vi "camera acquire test.vi"() -> ()   [LabVIEW 2014]
uses:
  SubVIs/ctt's/Image size and binning.ctl
  SubVIs/ctt's/Camera Setup Acquisition.ctl
panel:
  in  "EM CCD Gain":u16(slide)=300 scale=0.01..300.0
  in  "Acquisition Parameters":T1={"Set Acquisition Mode"=enum."Run till abort", "Trigger Mode"=enum."Internal", "Set VS Speed"=6.5, "Pixel Rate"=enum."EM CCD 5 Mhz 14 bits", "V Shift Amplitude"=enum."normal", "Readout Mode"=enum."Image", "Single Track \nSettings"={"centre"=0, "height"=1}, "Preamp Gain"=enum."2.4", "Number of\nAccumulations"=1, "Number of Kinetics"=1, "Accumulation\nCycle (s)"=1.0, "Kinetic Cycle Time (s)"=0.0, "High Capacity?"=FALSE} {"Single Track \nSettings"."centre" min=0 max=1024; "Single Track \nSettings"."height" min=1 max=1024; "Set VS Speed" min=0.0 format="%#_2f"}
  in  "Image Size":T2 {"V Bin" min=0.0; "H Bin" min=0.0 step=1.0}
  out "Error Out":errorcluster
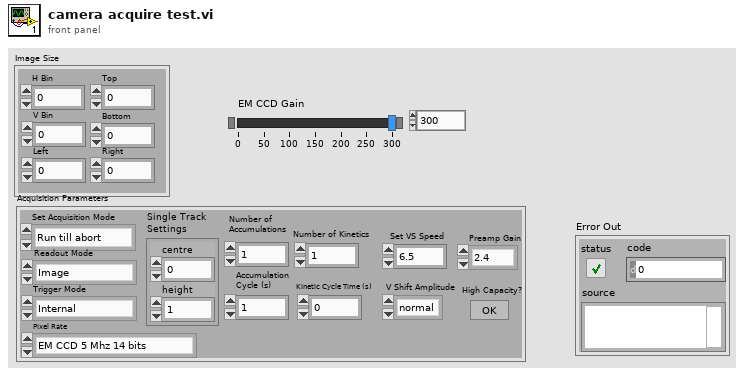
[diagram p1: front panel]
types:
  T1 = typedef "Camera Setup Acquisition.ctl" = cluster{"Set Acquisition Mode":enum16{"(do nothing)", "Single Scan", "Accumulate", "Kinetics", "Fast Kinetics", "Run till abort"}, "Trigger Mode":enum16{"Internal", "External"}, "Set VS Speed":dbl, "Pixel Rate":enum16{"EM CCD 10 Mhz 14 bits", "EM CCD 5 Mhz 14 bits", "EM CCD 3 Mhz 14 bits", "EM CCD 1 Mhz 16 bits", "Standard CCD 3 Mhz 14 bits", "Standard CCD 1 Mhz 16 bits"}, "V Shift Amplitude":enum16{"normal", "+1", "+2", "+3", "+4"}, "Readout Mode":enum16{"Full Vertical Binning", "Multi-Track", "Random-Track", "Single-Track", "Image"}, "Single Track \nSettings":cluster{"centre":i32, "height":i32}, "Preamp Gain":enum16{"1.0", "2.4", "5.0"}, "Number of\nAccumulations":i32, "Number of Kinetics":i32, "Accumulation\nCycle (s)":dbl, "Kinetic Cycle Time (s)":dbl, "High Capacity?":bool}
  T2 = typedef "Image size and binning.ctl" = cluster{"H Bin":dbl, "V Bin":dbl, "Left":dbl, "Right":dbl, "Top":dbl, "Bottom":dbl}
  T3 = typedef "Image Type" = u32
  T4 = typedef "IMAQ Image.ctl" = refnum<image>
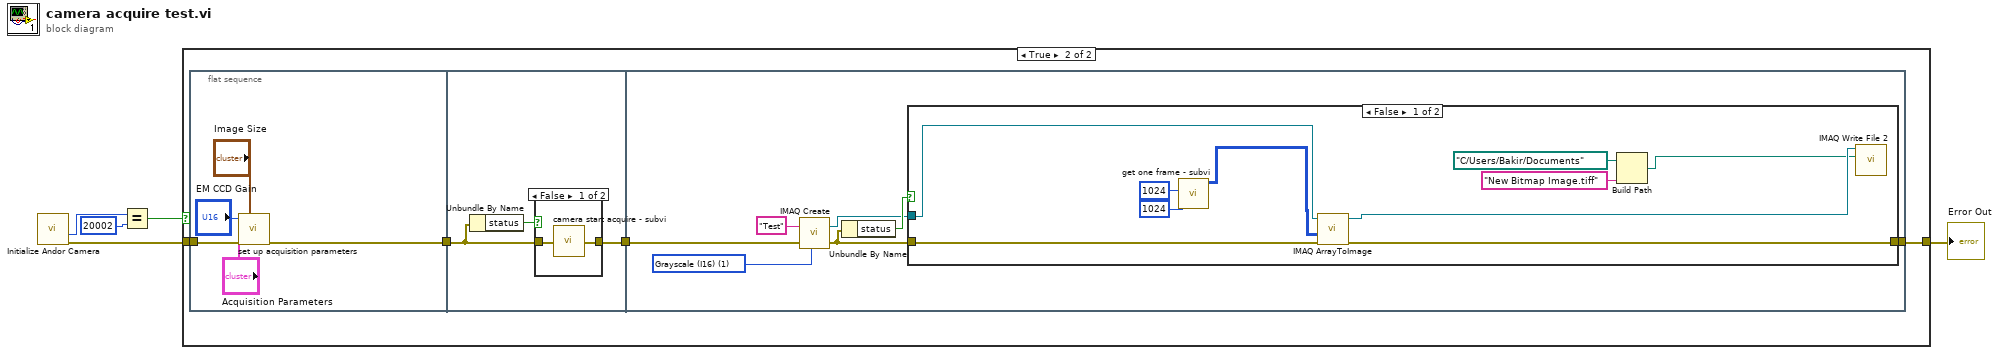
[diagram p0: block diagram]
diagram:
  n1 = call "Initialize Andor Camera.vi"() -> ("Error Out 2"=w4:errorcluster, "Drv Success?"=w1:i32)  [unwired: 10 in]
  n2 = Equal?(x=w1, y=20002) -> (x = y?=w3:bool)
  n3 = case shown="True" w3 {
    tunnel: [w6 w8] -> w5
    tunnel: w4 -> [w6 w7]
    frame False {
    }
    frame True {
      n4 = flat-sequence {
        tunnel: [w14] -> w10
        tunnel: w7 -> [w15]
        tunnel: w10 -> [w17]
        tunnel: [w16] -> w9
        tunnel: w9 -> [w25]
        tunnel: [w22] -> w8
        frame #0 {
          n5 = call "set up acquisition parameters.vi"("error in (no error)"=w15, "Acquisition Parameters"="Acquisition Parameters", "Image Size"="Image Size", "EM CCD Gain"="EM CCD Gain") -> ("error out"=w14:errorcluster)  [unwired: 2 in, 2 out]
        }
        frame #1 {
          n6 = Unbundle By Name(w17) -> ("status"=w18:bool)
          n7 = case shown="False" w18 {
            tunnel: w17 -> [w20 w21]
            tunnel: [w19 w21] -> w16
            frame False {
              n8 = call "camera start acquire - subvi.vi"("error in"=w20) -> ("error out"=w19:errorcluster)
            }
            frame True {
            }
          }
        }
        frame #2 {
          w27 = T3 1 items=["Grayscale (U8)", "Grayscale (I16)", "Grayscale (SGL)", "Complex (CSG)", "RGB (U32)", "HSL (U32)", "RGB (U64)", "Grayscale (U16)"] ("Image Type")
          n9 = call "IMAQ Create"("Image Name"="Test", "Image Type"=w27, "error in (no error)"=w25) -> ("New Image"=w24:T4, "error out"=w23:errorcluster)  [unwired: 2 in]
          n10 = Unbundle By Name(w23) -> ("status"=w28:bool)
          n11 = case shown="False" w28 {
            tunnel: w23 -> [w32 w39]
            tunnel: w24 -> [w38 _]
            tunnel: [w37 w39] -> w22
            frame False {
              n12 = call "get one frame - subvi.vi"("Image Height"=1024, "Image Width"=1024) -> ("Image Array"=w29:i32[][])  [unwired: 9 in]
              n13 = call "IMAQ ArrayToImage"("error in (no error)"=w32, "Image Pixels (I16)"=w29, "Image"=w38) -> ("error out"=w37:errorcluster, "Image Out"=w36:T4)  [unwired: 3 in, 4 out]
              n14 = Build Path(base path=path "C:/Users/Bakir/Documents", name or relative path="New Bitmap Image.tiff") -> (appended path=w35:path)
              n15 = call-poly "IMAQ Write File 2"("File Path"=w35, "Image"=w36) -> ()  [unwired: 8 in, 2 out]
            }
            frame True {
            }
          }
        }
      }
    }
  }
  "Error Out" <- w5
